vi "Action Single Trigger.vi"(8 "error in (no error)":errorcluster, 11 "PM-EMP in":refnum<class "PM-EMP.lvclass">) -> (0 "error out":errorcluster, 3 "PM-EMP out":refnum<class "PM-EMP.lvclass">)   [LabVIEW 2020, in "PM-EMP.lvclass"]
uses:
  PM-EMP.lvclass
  C:/Sandbox/Git_Sandbox/WiSpry Test Framework source code (LV20)/WiSpry Test Framework/Instruments/Instrument.lvclass
  Instrument.lvclass/Instrument.ctl
  Instrument.lvclass
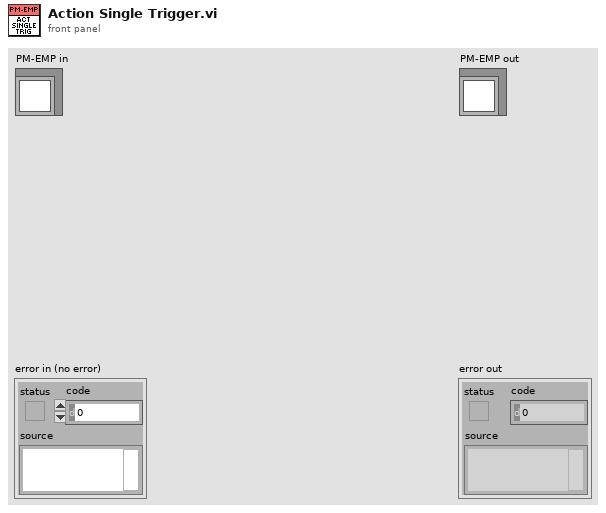
[diagram p1: front panel]
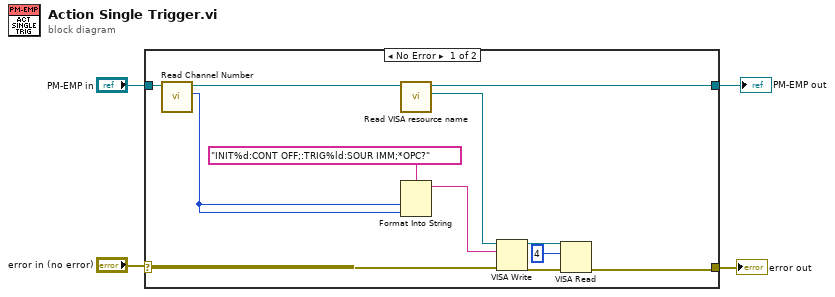
[diagram p0: block diagram]
diagram:
  n1 = case shown="No Error" "error in (no error)" {
    selector: "error in (no error)" -> [w16 w18]
    tunnel: [w8 w18] -> w3
    tunnel: "PM-EMP in" -> [w7 w17]
    tunnel: [w14 w17] -> w1
    frame No Error {
      n2 = call-dynamic "Read Channel Number.vi"("Power Meter in"=w7) -> ("Channel Number"=w5:u8, "Power Meter out"=w6:refnum<class "PM-EMP.lvclass">)  [unwired: 9 in]
      n3 = call "Read VISA resource name.vi"("Instrument in"=w6) -> ("VISA resource name"=w15:refnum<visa-resource-name>, "Instrument out"=w14:refnum<class "PM-EMP.lvclass">)  [unwired: 9 in]
      n4 = Format Into String(format string="INIT%d:CONT OFF;:TRIG%ld:SOUR IMM;*OPC?", w5, w5) -> (resulting string=w12:string)  [unwired: 2 in, 1 out]
      n5 = VISA Write(VISA resource name=w15, write buffer=w12, error in (no error)=w16) -> (VISA resource name out=w10:refnum<visa-resource-name>, error out=w11:errorcluster)  [unwired: 1 out]
      n6 = VISA Read(VISA resource name=w10, byte count=u32 4, error in (no error)=w11) -> (error out=w8:errorcluster)  [unwired: 3 out]
    }
    frame Error {
    }
  }
  "error out" <- w3
  "PM-EMP out" <- w1
